vi "Configure Trigger (Parallel).vi"(0 "VISA resource name":refnum<visa-resource-name>, 5 "Trigger Source (1: Bus 1)":u16(ring)=1 items=["Bus 1"=1, "Bus 2"=2, "Bus 3"=3, "Bus 4"=4], 9 "Data Value (XXXXXXXX)":string="XXXXXXXX", 11 "error in (no error)":errorcluster) -> (4 "VISA resource name out":refnum<visa-resource-name>, 15 "error out":errorcluster)   [LabVIEW 2016, in "Tektronix DPO MSO 2000 4000 Series.lvlib"]
doc: "Configures Parallel trigger settings for the oscilloscope."
uses:
  Tektronix DPO MSO 2000 4000 Series.lvlib
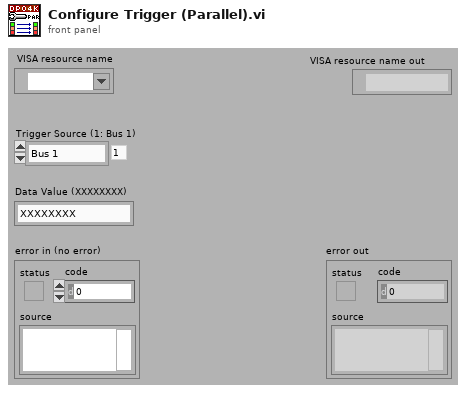
[diagram p1: front panel]
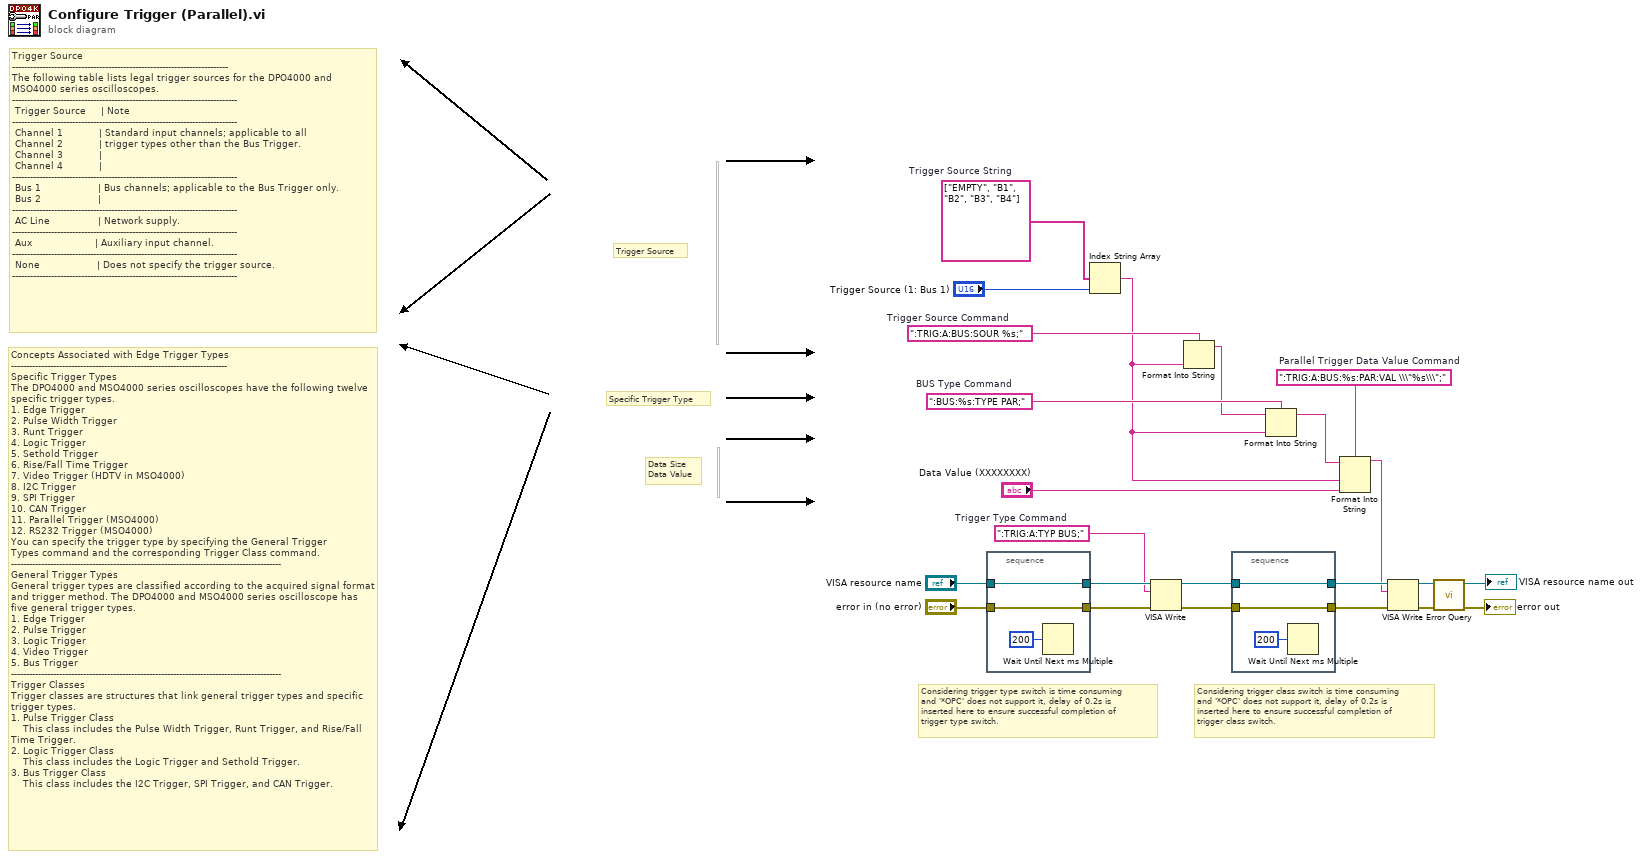
[diagram p0: block diagram]
diagram:
  w5 = ":TRIG:A:BUS:%s:PAR:VAL \\\"%s\\\";"  # Parallel Trigger Data Value Command
  w18 = string[] ["EMPTY", "B1", "B2", "B3", "B4"]  # Trigger Source String
  w16 = ":TRIG:A:BUS:SOUR %s;"  # Trigger Source Command
  w17 = ":BUS:%s:TYPE PAR;"  # BUS Type Command
  w21 = ":TRIG:A:TYP BUS;"  # Trigger Type Command
  # "Concepts Associated with Edge Trigger Types\n------------------------------------------------------------------------\nSpecific Trigger Types\nThe DPO4000 and MSO4000 series oscilloscopes have the following twelve specific trigger types.\n1. Edge Trigger\n2. Pulse Width Trigger\n3. Runt Trigger\n4. Logic Trigger\n5. Sethold Trigger\n6. Rise/Fall Time Trigger\n7. Video Trigger (HDTV in MSO4000)\n8. I2C Trigger\n9. SPI Trigger\n10. CAN Trigger\n11. Parallel Trigger (MSO4000)\n12. RS232 Trigger (MSO4000)\nYou can specify the trigger type by specifying the General Trigger \nTypes command and the corresponding Trigger Class command.\n------------------------------------------------------------------------------------------\nGeneral Trigger Types \nGeneral trigger types are classified according to the acquired signal format and trigger method. The DPO4000 and MSO4000 series oscilloscope has five general trigger types.\n1. Edge Trigger\n2. Pulse Trigger\n3. Logic Trigger\n4. Video Trigger\n5. Bus Trigger\n------------------------------------------------------------------------------------------\nTrigger Classes\nTrigger classes are structures that link general trigger types and specific trigger types.\n1. Pulse Trigger Class\n    This class includes the Pulse Width Trigger, Runt Trigger, and Rise/Fall Time Trigger.\n2. Logic Trigger Class\n    This class includes the Logic Trigger and Sethold Trigger.\n3. Bus Trigger Class\n    This class includes the I2C Trigger, SPI Trigger, and CAN Trigger."
  # "Trigger Source\n------------------------------------------------------------------------\nThe following table lists legal trigger sources for the DPO4000 and MSO4000 series oscilloscopes.\n---------------------------------------------------------------------------\n Trigger Source     | Note                                                           \n---------------------------------------------------------------------------\n Channel 1            | Standard input channels; applicable to all      \n Channel 2            | trigger types other than the Bus Trigger.         \n Channel 3            |     \n Channel 4            |\n---------------------------------------------------------------------------\n Bus 1                   | Bus channels; applicable to the Bus Trigger only.\n Bus 2                   | \n---------------------------------------------------------------------------\n AC Line                | Network supply.\n---------------------------------------------------------------------------\n Aux                     | Auxiliary input channel.\n---------------------------------------------------------------------------\n None                   | Does not specify the trigger source.\n---------------------------------------------------------------------------"
  # "Considering trigger class switch is time consuming\nand '*OPC' does not support it, delay of 0.2s is \ninserted here to ensure successful completion of\ntrigger class switch."
  # "Data Size\nData Value"
  # "Specific Trigger Type"
  # "Trigger Source"
  # "Considering trigger type switch is time consuming\nand '*OPC' does not support it, delay of 0.2s is \ninserted here to ensure successful completion of\ntrigger type switch."
  n1 = stacked-sequence {
    tunnel: "VISA resource name" -> [w25]
    tunnel: [w25] -> w23
    tunnel: "error in (no error)" -> [w24]
    tunnel: [w24] -> w22
    frame #0 {
      n2 = Wait Until Next ms Multiple(millisecond multiple=u32 200) -> ()  [unwired: 1 out]
    }
  }
  n3 = Index String Array(1:"Trigger Source (1: Bus 1)", 2:w18) -> (0:w3:string)  [unwired: 1 in]
  n4 = VISA Write(VISA resource name=w23, write buffer=w21, error in (no error)=w22) -> (VISA resource name out=w20:refnum<visa-resource-name>, error out=w19:errorcluster)  [unwired: 1 out]
  n5 = Format Into String(format string=w16, w3) -> (resulting string=w15:string)  [unwired: 2 in, 1 out]
  n6 = stacked-sequence {
    tunnel: w20 -> [w28]
    tunnel: [w28] -> w14
    tunnel: w19 -> [w27]
    tunnel: [w27] -> w13
    frame #0 {
      n7 = Wait Until Next ms Multiple(millisecond multiple=u32 200) -> ()  [unwired: 1 out]
    }
  }
  n8 = Format Into String(format string=w17, initial string=w15, w3) -> (resulting string=w2:string)  [unwired: 1 in, 1 out]
  n9 = Format Into String(format string=w5, initial string=w2, w3, "Data Value (XXXXXXXX)") -> (resulting string=w6:string)  [unwired: 1 in, 1 out]
  n10 = VISA Write(VISA resource name=w14, write buffer=w6, error in (no error)=w13) -> (VISA resource name out=w12:refnum<visa-resource-name>, error out=w11:errorcluster)  [unwired: 1 out]
  n11 = call "Error Query.vi"("error in (no error)"=w11, "VISA resource name"=w12) -> ("error out"=→"error out":errorcluster, "VISA resource name out"=→"VISA resource name out":refnum<visa-resource-name>)  [unwired: 6 in, 2 out]
